vi "log_test.vi"   [LabVIEW 2015, in "pcfs_hdf5_log.lvclass"]
uses:
  pcfs_hdf5_log.lvclass
  Detector_Class/Picoquant/Hydraharp/hydraharp_panel/hpanel_acq_modes.ctl
  lvoop_dll-master/picoquant_Tmodes.ctl
types:
  T1 = typedef "picoquant_Tmodes.ctl" = u16
  T2 = typedef "hpanel_acq_modes.ctl" = u16
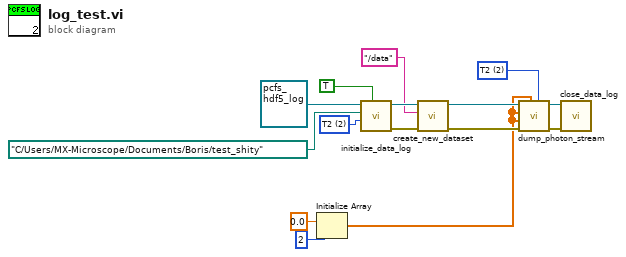
[diagram p0: block diagram]
diagram:
  w4 = T1 2 items=["T2"=2, "T3"=3] ("acq_mode")
  w12 = T2 2 items=["T2"=2, "T3"=3] ("Mode")
  n1 = Initialize Array(0.0 ("element"), 2 ("dimension size")) -> (w1:dbl[])
  n2 = call-dynamic "initialize_data_log.vi"("Overwrite?"=TRUE, "Initialization Data"=w12, "Path"=path "C:/Users/MX-Microscope/Documents/Boris/test_shity", "pcfs_hdf5_log in"=refnum<class "pcfs_hdf5_log.lvclass"> refnum) -> ("error out"=w9:errorcluster, "pcfs_hdf5_log out"=w11:refnum<class "pcfs_hdf5_log.lvclass">)  [unwired: 6 in]
  n3 = call-dynamic "create_new_dataset.vi"("error in (no error)"=w9, "Path"="/data", "pcfs_hdf5_log in"=w11) -> ("error out"=w8:errorcluster, "pcfs_hdf5_log out"=w7:refnum<class "pcfs_hdf5_log.lvclass">)  [unwired: 7 in]
  n4 = call-dynamic "dump_photon_stream.vi"("Ring"=w4, "sync"=w1, "error in (no error)"=w8, "channels"=w1, "photon_records"=w1, "pcfs_hdf5_log in"=w7) -> ("error out"=w5:errorcluster, "pcfs_hdf5_log out"=w6:refnum<class "pcfs_hdf5_log.lvclass">)  [unwired: 4 in]
  n5 = call-dynamic "close_data_log.vi"("error in (no error)"=w5, "pcfs_hdf5_log in"=w6) -> ()  [unwired: 8 in, 2 out]
